vi "fine approach Pico.vi"(7 "Boolean":bool, 8 "error in":errorcluster, 9 "Z Voltage (V)":i16, 10 "pico step":i16, 11 "Coarse Approach.lvclass":refnum<class "Coarse Approach.lvclass">) -> (0 "error out":errorcluster, 2 "Is moving?":bool, 3 "Coarse Approach.lvclass":refnum<class "Coarse Approach.lvclass">)   [LabVIEW 2020, in "Coarse Approach.lvclass"]
uses:
  Coarse Approach.lvclass
  Coarse Approach.lvclass/Coarse Approach.ctl
  PI P123.01 & PiezoDrive TD250 & NI USB 7855R/PI P123.01 & PiezoDrive TD250 & NI USB 7855R.lvclass
  Newport Model 8742/New Focus Model 8742.lvclass
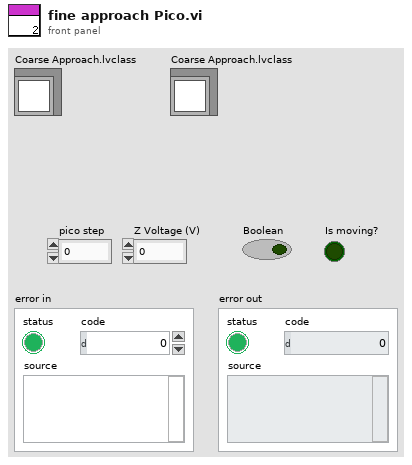
[diagram p1: front panel]
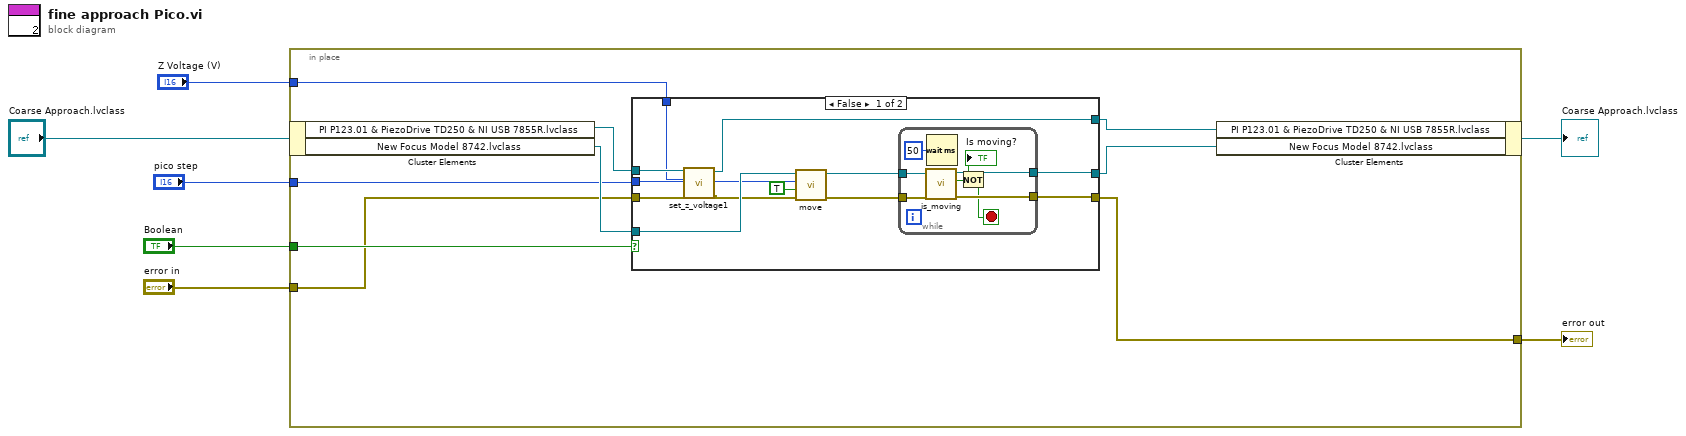
[diagram p0: block diagram]
diagram:
  n1 = in-place {
    in-place-border: "Boolean" -> [w16]
    in-place-border: "error in" -> [w13]
    in-place-border: "pico step" -> [w10]
    in-place-border: "Z Voltage (V)" -> [w9]
    in-place-border: [w8] -> w1
    n2 = in-place-cluster #1("Coarse Approach.lvclass") -> ("PI P123.01 & PiezoDrive TD250 & NI USB 7855R.lvclass"=w15:refnum<class "PI P123.01 & PiezoDrive TD250 & NI USB 7855R.lvclass">, "New Focus Model 8742.lvclass"=w14:refnum<class "New Focus Model 8742.lvclass">)
    n3 = case shown="False" w16 {
      tunnel: w14 -> [w27 w38]
      tunnel: [w19 w38] -> w11
      tunnel: w13 -> [w25 w36]
      tunnel: w15 -> [w26 w37]
      tunnel: [w24 w37] -> w12
      tunnel: w10 -> [w23 _]
      tunnel: w9 -> [w22 _]
      tunnel: [w18 w36] -> w8
      frame False {
        n4 = call "set_z_voltage1.vi"("error in (no error)"=w25, "Z Voltage (V)"=w22, "PI P123.01 & PiezoDrive TD250 & NI USB 7855R in"=w26) -> ("error out"=w17:errorcluster, "PI P123.01 & PiezoDrive TD250 & NI USB 7855R out"=w24:refnum<class "PI P123.01 & PiezoDrive TD250 & NI USB 7855R.lvclass">)  [unwired: 7 in]
        n5 = call "move.vi"("error in"=w17, "Relative? (T)"=TRUE, "Destination (steps)"=w23, "Newport Model 8742 in"=w27) -> ("error out"=w21:errorcluster, "Newport Model 8742 out"=w20:refnum<class "New Focus Model 8742.lvclass">)  [unwired: 6 in]
        n6 = while {
          tunnel: [w34] -> w18
          tunnel: w21 -> [w33]
          tunnel: w20 -> [w32]
          tunnel: [w31] -> w19
          stop <- w30 stop-if-true
          n7 = call "is_moving.vi"("error in"=w33, "Newport Model 8742 in"=w32) -> ("error out"=w34:errorcluster, "Is moving?"=w35:bool, "Newport Model 8742 out"=w31:refnum<class "New Focus Model 8742.lvclass">)  [unwired: 7 in]
          "Is moving?" <- w35
          n8 = Wait (ms)(milliseconds to wait=u32 50) -> ()  [unwired: 1 out]
          n9 = Not(x=w35) -> (.not. x?=w30:bool)
        }
      }
      frame True {
      }
    }
    n10 = in-place-cluster #1("PI P123.01 & PiezoDrive TD250 & NI USB 7855R.lvclass"=w12, "New Focus Model 8742.lvclass"=w11) -> (→"Coarse Approach.lvclass":refnum<class "Coarse Approach.lvclass">)
  }
  "error out" <- w1
